vi "Run Test - Station Selection (SubVI).vi"(8 "error in (no error)":errorcluster, 10 "Current Station":string, 11 "Station Names":string[](array[string])) -> (0 "error out":errorcluster, 2 "Cancel out":bool, 3 "Station":string)   [LabVIEW 2019]
panel:
  in  "Cancel":bool
  in  "Ok":bool
  in  "Select station to change":i32(listbox)
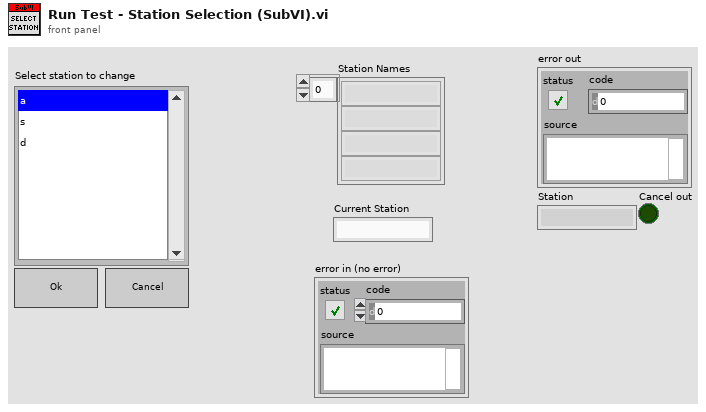
[diagram p1: front panel]
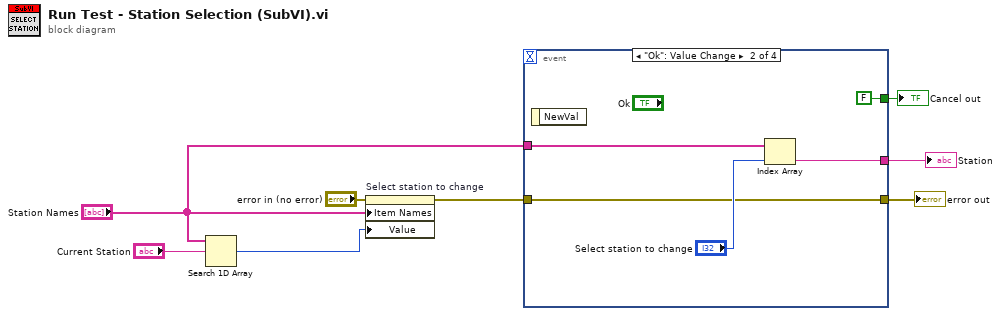
[diagram p0: block diagram]
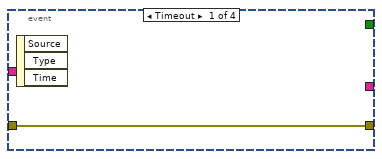
[diagram p2: hidden frame]
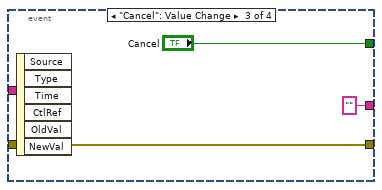
[diagram p3: hidden frame]
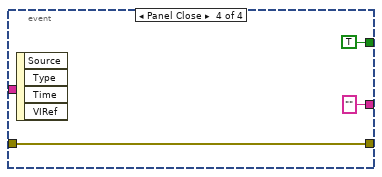
[diagram p4: hidden frame]
diagram:
  n1 = Search 1D Array(1D array="Station Names", element="Current Station") -> (index of element=w8:i32)  [unwired: 1 in]
  n2 = property on="Select station to change" class="LstBox (strict)"(error in="error in (no error)", "Item Names"="Station Names", "Value"=w8) -> (error out=w5:errorcluster)  [unwired: 1 in, 1 out]
  n3 = event shown="[1] \"Ok\": Value Change" {
    selector: _ -> [_ _ _ _]
    dyn-events: _ -> [_ _ _ _]
    timeout: _ -> [_ _ _ _]
    tunnel: w5 -> [w9 w10 w15 w18]
    tunnel: "Station Names" -> [_ w14 _ _]
    tunnel: [_ w12 "" ""] -> w3
    tunnel: [_ FALSE ("Cancel") "Cancel" TRUE ("Cancel")] -> w2
    tunnel: [w9 w10 w15 w18] -> w1
    event Timeout {
      n4 = event-data() -> ()  [unwired: 1 in, 3 out]
    }
    event "Ok": Value Change {
      n5 = event-data() -> ()  [unwired: 1 in, 1 out]
      n6 = Index Array(array=w14, index="Select station to change") -> (element=w12:string)
    }
    event "Cancel": Value Change {
      n7 = event-data() -> ()  [unwired: 1 in, 6 out]
    }
    event Panel Close {
      n8 = event-data() -> ()  [unwired: 1 in, 4 out]
    }
  }
  "error out" <- w1
  "Station" <- w3
  "Cancel out" <- w2
